vi "Draw Cross.vi"(1 "Color":u32(colorbox)=16711680, 2 "Cross Size":dbl, 3 "Cluster":cluster{"Center X":dbl, "Center Y":dbl}, 4 "Image":T1) -> (0 "Image Out":T1)   [LabVIEW 2013]
uses:
  <vilib>/vision/Image Controls.llb/IMAQ Image.ctl
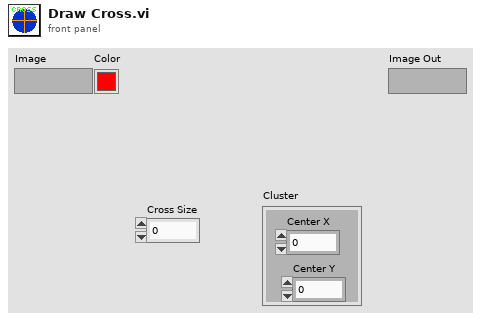
[diagram p1: front panel]
types:
  T1 = typedef "IMAQ Image.ctl" = refnum<image>
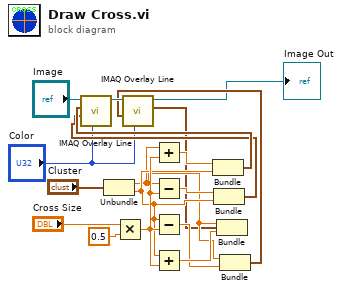
[diagram p0: block diagram]
diagram:
  n1 = Unbundle("Cluster") -> ("Center X"=w6:dbl, "Center Y"=w10:dbl)
  n2 = Multiply(x="Cross Size", y=0.5) -> (x*y=w13:dbl)
  n3 = Add(x=w6, y=w13) -> (x+y=w12:dbl)
  n4 = Subtract(x=w6, y=w13) -> (x-y=w9:dbl)
  n5 = Subtract(x=w10, y=w13) -> (x-y=w5:dbl)
  n6 = Add(x=w10, y=w13) -> (x+y=w7:dbl)
  n7 = Bundle(w12, "Center Y"=w10) -> (w11:cluster{dbl, "Center Y":dbl})  [unwired: 1 in]
  n8 = Bundle(w9, "Center Y"=w10) -> (w8:cluster{dbl, "Center Y":dbl})  [unwired: 1 in]
  n9 = call "IMAQ Overlay Line"("Color"="Color", "End Point"=w8, "Start Point"=w11, "Image"="Image") -> ("Image Out"=w18:T1)  [unwired: 6 in, 1 out]
  n10 = Bundle("Center X"=w6, w7) -> (w3:cluster{"Center X":dbl, dbl})  [unwired: 1 in]
  n11 = Bundle("Center X"=w6, w5) -> (w4:cluster{"Center X":dbl, dbl})  [unwired: 1 in]
  n12 = call "IMAQ Overlay Line"("Color"="Color", "End Point"=w4, "Start Point"=w3, "Image"=w18) -> ("Image Out"=→"Image Out":T1)  [unwired: 6 in, 1 out]
